vi "AlliGator Preprocess Decay v3.vi"(6 "Decay Preprocessing Parameters":T1={"Background Subtraction"=FALSE, "Straighten Decay"=FALSE, "Reverse Gates"=FALSE, "1-Normalized Decay"=FALSE, "Smoothen Decay"=FALSE, "Smoothing Parameter"=0.0, "Shift Decay"=FALSE, "Decay Shift Parameters"={"Type"=enum."Default", "Shift"=0.0, "Threshold"=0.0, "Rotate"=FALSE}, "Extrapolate Decay"=FALSE, "Additional Points"=0, "Head Fraction"=0.0, "Pixel-Normalize Decay"=FALSE, "Use Periodicity"=FALSE, "Use Cursors"=FALSE, "Tail Fraction"=0.0, "Use Decay Pre-Processing"=TRUE, "Fold Decay"=FALSE, "# Folds"=1, "[0-1]-Normalized Decay"=FALSE} {"# Folds" min=1}, 8 "Error In":errorcluster, 9 "Time-Gated Reference Decay":cluster{"t Array":dbl[], "I Array":dbl[]}, 10 "# Pixels":i32=1, 11 "Decay (in)":T9) -> (0 "Error Out":errorcluster, 3 "Decay (out)":T9, 5 "Decay Metadata":T4={"ROI Descriptor"={"Global Rectangle"=[], "Contours"=[]}, "ROI Center"={"X"=0, "Y"=0}, "Decay Background Subtraction Info"={"Laser Period"=0.0, "Gate Duration"=0.0, "Baseline Subtraction Method"=enum."Mean", "Background Definition Range"={"Min Gate"=0.0, "Max Gate"=0.0}, "Total Intensity w/o Bkgd Subtraction"=0.0, "Bkgd-subtracted Intensity (exp)"=0.0, "# Data Points"=0, "Background/Gate"=0.0, "Fitted Lifetime"=0.0, "Bkgd-subtracted Intensity (theo)"=0.0}, "Decay Reverted"=FALSE, "Decay Smoothened"=FALSE, "Decay Straightened"=FALSE, "Fitted Tau (Decay Straightening)"=0.0, "Decay Shift Parameters"={"Type"=enum."Default", "Shift"=0.0, "Threshold"=0.0, "Rotate"=FALSE}, "Decay Shifted"=FALSE, "Decay Extrapolated"=FALSE, "Decay Extrapolation Parameters"={"Additional Points"=0, "Head Fraction"=0.0, "Fitted Tau"=0.0, "Use Periodicity"=FALSE, "Use Cursors"=FALSE, "Tail Fraction"=0.0}, "Decay Normalized"=FALSE, "Fold Decay"=FALSE, "# Folds"=1} {"# Folds" min=1; "ROI Descriptor"."Contours"."Type" items=["No Selection", "Point", "Line", "Rectangle", "Oval", "Polygon", "Freehand Region", "Annulus", "Unused2", "Unused3", "Broken Line", "Freehand Line", "Rotated Rectangle"]}, 7 "Message":string)   [LabVIEW 2021, in "AlliGator Decay Analysis.lvlib" / "AlliGator Decay Preprocessing.lvlib"]
doc: "Applies the different selected pre-processing steps on the provided decay in the specified order."
uses:
  AlliGator Decay Preprocessing.lvlib
  AlliGator Decay Metadata v3.ctl
  AlliGator Decay Background Subtraction Info.ctl
  AlliGator Baseline Subtraction Method.ctl
  Graphs/XY Graph/XY Graph Plot Shift Parameters.ctl
  Graphs/XY Graph/XY Graph Plot Shift Method.ctl
  AlliGator Decay Extrapolation Parameters.ctl
  AlliGator Decay Preprocessing Parameters.ctl
  AlliGator Settings List.ctl
  AlliGator Decay Preprocessing Steps.ctl
  Variant/Variant to Data/Variant to Boolean.vi
  <vilib>/Utility/error.llb/Error Cluster From Error Code.vi
  Variant/Variant to Data/Variant to [String].vi
  <vilib>/ErrorRing/Error Ring.xnode
  AlliGator Settings.lvlib
  Variant/Variant to Data/Variant to Data.lvlib
  Graphs/XY Graph/XY Graph Add-Ons.lvlib
  AlliGator Phasor Graph.lvlib
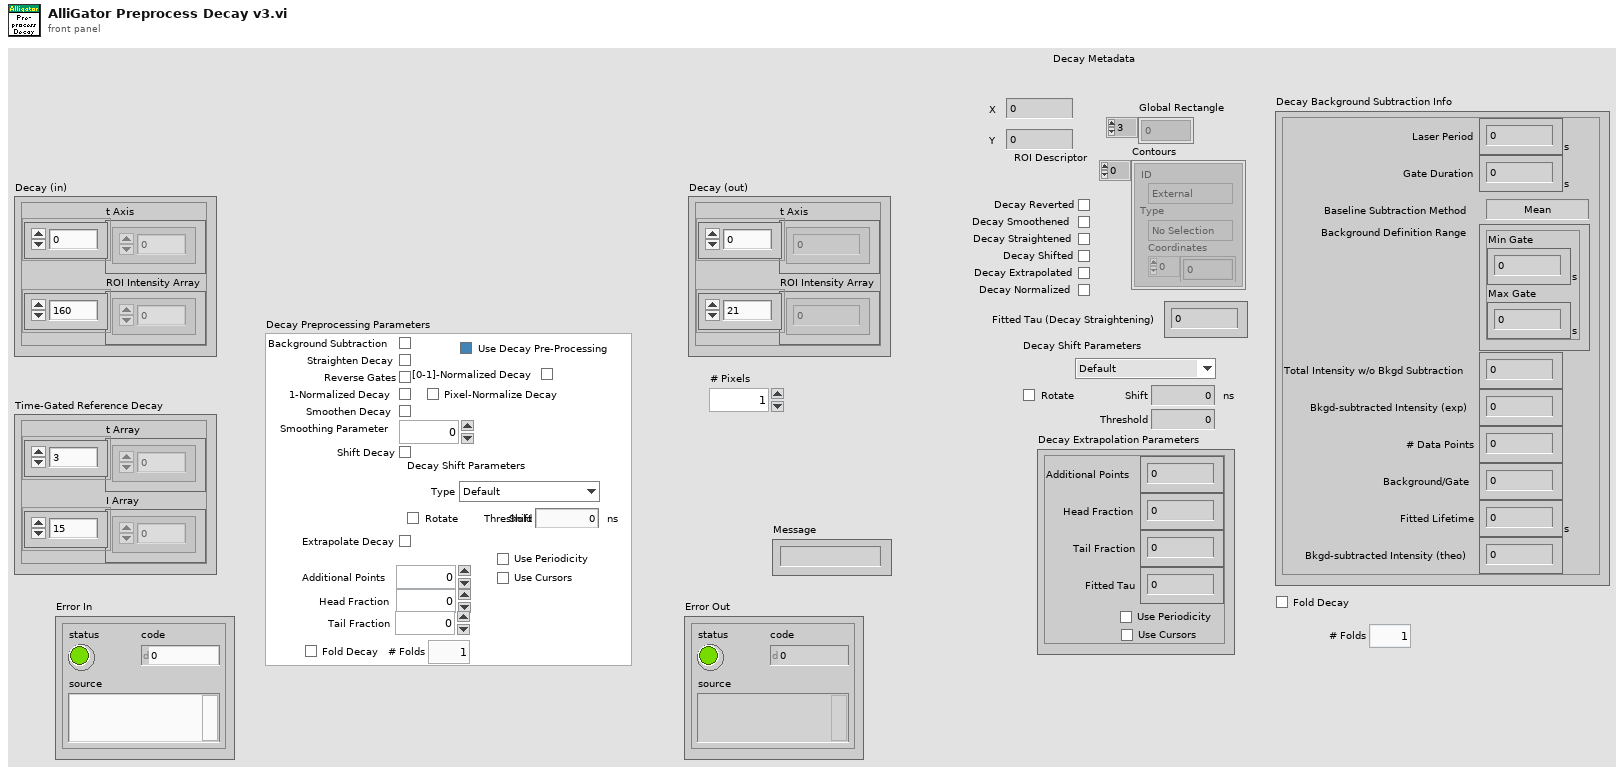
[diagram p1: front panel]
types:
  T1 = typedef "AlliGator Decay Analysis.lvlib/AlliGator Decay Preprocessing.lvlib/AlliGator Decay Preprocessing Parameters.ctl" = cluster{"Background Subtraction":bool, "Straighten Decay":bool, "Reverse Gates":bool, "1-Normalized Decay":bool, "Smoothen Decay":bool, "Smoothing Parameter":dbl, "Shift Decay":bool, "Decay Shift Parameters":T2, "Extrapolate Decay":bool, "Additional Points":u32, "Head Fraction":dbl, "Pixel-Normalize Decay":bool, "Use Periodicity":bool, "Use Cursors":bool, "Tail Fraction":dbl, "Use Decay Pre-Processing":bool, "Fold Decay":bool, "# Folds":u32, "[0-1]-Normalized Decay":bool}
  T2 = typedef "XY Graph Add-Ons.lvlib/XY Graph Plot Shift Parameters.ctl" = cluster{"Type":T3, "Shift":dbl[unit], "Threshold":dbl, "Rotate":bool}
  T3 = typedef "XY Graph Add-Ons.lvlib/XY Graph Plot Shift Method.ctl" = enum16{"Default", "CFD", "Threshold", "Cross-Correlation"}
  T4 = typedef "AlliGator Phasor Graph.lvlib/AlliGator Decay Metadata v3.ctl" = cluster{"ROI Descriptor":T5, "ROI Center":cluster{"X":i32, "Y":i32}, "Decay Background Subtraction Info":T6, "Decay Reverted":bool, "Decay Smoothened":bool, "Decay Straightened":bool, "Fitted Tau (Decay Straightening)":dbl, "Decay Shift Parameters":T2, "Decay Shifted":bool, "Decay Extrapolated":bool, "Decay Extrapolation Parameters":T8, "Decay Normalized":bool, "Fold Decay":bool, "# Folds":u32}
  T5 = typedef "ROI Descriptor" = cluster{"Global Rectangle":i32[], "Contours":cluster{"ID":enum32{"External", "Internal"}, "Type":u32, "Coordinates":i32[]}[]}
  T6 = typedef "AlliGator Decay Analysis.lvlib/AlliGator Decay Preprocessing.lvlib/AlliGator Decay Background Subtraction Info.ctl" = cluster{"Laser Period":dbl[unit], "Gate Duration":dbl[unit], "Baseline Subtraction Method":T7, "Background Definition Range":cluster{"Min Gate":dbl[unit], "Max Gate":dbl[unit]}, "Total Intensity w/o Bkgd Subtraction":dbl, "Bkgd-subtracted Intensity (exp)":dbl, "# Data Points":i32, "Background/Gate":dbl, "Fitted Lifetime":dbl[unit], "Bkgd-subtracted Intensity (theo)":dbl}
  T7 = typedef "AlliGator Decay Analysis.lvlib/AlliGator Decay Preprocessing.lvlib/AlliGator Baseline Subtraction Method.ctl" = enum16{"Mean", "Min", "Square Gated Single-Exponential", "File", "Constant"}
  T8 = typedef "AlliGator Decay Analysis.lvlib/AlliGator Decay Preprocessing.lvlib/AlliGator Decay Extrapolation Parameters.ctl" = cluster{"Additional Points":u32, "Head Fraction":dbl, "Fitted Tau":dbl, "Use Periodicity":bool, "Use Cursors":bool, "Tail Fraction":dbl}
  T9 = cluster{"t Axis":dbl[], "ROI Intensity Array":dbl[]}
  T10 = typedef "AlliGator Settings.lvlib/AlliGator Settings List.ctl" = enum16{"GUI:Visible Settings Tab", "GUI:Last Run Version", "Source Image:Use Image Histogram for Contrast", "Source Image:Low Count Pixels Rejection Options", "Source Image:High Count Pixels Rejection Options", "Source Image:Use Image Brightness", "Source Image:Blend Overlay with Image Background", "Source Image:Use Fixed ROI Diameter", "Source Image:ROI Diameter", "Source Image:ROI Center Color", "Source Image:Peak Threshold", "Source Image:Intensity Threshold", "Source Image:Image Binning Options", "Source Image:Image Smoothing Options", "Source Image:Image Histogram Active", "Source Image:Invert Binary Mask", "Source Image:Hot Pixel Removal", "Source Image:Overlay Analyzed ROI Center", "Source Image:Auto-Adjust Contrast", "Source Image:Histogram Lower Percentile", "Source Image:Histogram Upper Percentile", "Source Image:Save Source Image", "Source Image:Scale Bar Options", "Source Image:Image Resolution (Pixel Size)", "Source Image:Flatfield Correction", "Source Image:Show Dead Left Columns Correction", "Source Image:Dead Left Columns Correction", "Source Image:Image Pre-Processing Operations Order", "Data Information:Gate Width", "Data Information:Nanotime Gate Separation", "Data Information:Macrotime Gate Separation", "Data Information:Gate Step", "Data Information:# Gates", "Data Information:Gate Image Exposure", "Data Information:Gate Image Integration", "Data Information:Gates to Skip", "Data Information:Gates to Keep", "Data Information:Define Gates to", "Data Information:Channel Name", "Data Information:Available Channel Names", "Data Information:Channel Arithmetic", "Data Information:Background File Subtraction", "Data Information:Background File", "Data Information:Background Scaling Factor", "Data Information:Background Pile-up Correction", "Data Information:Background Pixel Well Capacity", "Data Information:Laser Period", "Data Information:SYNC Period", "Data Information:Pile-up Correction", "Data Information:Pixel Well Capacity", "Data Information:Dataset Scaling Factor", "Fluorescence Decay_Decay Pre-Processing:Reverse Gates", "Fluorescence Decay_Decay Pre-Processing:Verbose Decay Pre-Processing", "Fluorescence Decay_Decay Pre-Processing:Use Decay Pre-Processing", "Fluorescence Decay_Decay Pre-Processing:Background Subtraction", "Fluorescence Decay_Decay Pre-Processing:Background Definition Range", "Fluorescence Decay_Decay Pre-Processing:Baseline Subtraction Method", "Fluorescence Decay_Decay Pre-Processing:Decay Pre-Processing Operations Order", "Fluorescence Decay_Decay Pre-Processing:Smoothing Parameter", "Fluorescence Decay_Decay Pre-Processing:Shift Decay", "Fluorescence Decay_Decay Pre-Processing:Decay Shift Parameters", "Fluorescence Decay_Decay Pre-Processing:Fold Decay", "Fluorescence Decay_Decay Pre-Processing:# Folds", "Fluorescence Decay_Decay Pre-Processing:1-Normalize Decay", "Fluorescence Decay_Decay Pre-Processing:[0-1]-Normalize Decay", "Fluorescence Decay_Decay Pre-Processing:Smoothen Decay", "Fluorescence Decay_Decay Pre-Processing:Extrapolate Decay", "Fluorescence Decay_Decay Pre-Processing:Use Periodicity", "Fluorescence Decay_Decay Pre-Processing:Use Cursors", "Fluorescence Decay_Decay Pre-Processing:Tail Fraction", "Fluorescence Decay_Decay Pre-Processing:Head Fraction", "Fluorescence Decay_Decay Pre-Processing:Additional Points", "Fluorescence Decay_Decay Pre-Processing:Straighten Decay", "Fluorescence Decay_Decay Pre-Processing:Constant Background", "Fluorescence Decay_Decay Pre-Processing:Pixel-Normalize Decay", "Fluorescence Decay_Advanced Analysis:Extract IRF instead of Decay", "Fluorescence Decay_Advanced Analysis:IRF Extraction Options", "Fluorescence Decay_Advanced Analysis:IRF Optimization Options", "Fluorescence Decay_Advanced Analysis:Square Pulse Options", "Fluorescence Decay_Advanced Analysis:IRF Order", "Fluorescence Decay_Advanced Analysis:IRF Time Constants", "Fluorescence Decay_Advanced Analysis:Wavelet Analysis Options", "Fluorescence Decay_Advanced Analysis:Average Lifetime Options", "Fluorescence Decay_Fit Options:Fit Options", "Fluorescence Decay_Fit Options:Use Legacy Fitting Approach", "Fluorescence Decay_Fit Options:Use Data Information Laser Period", "Fluorescence Decay_Fit Parameters:Displayed Fit Parameters", "Fluorescence Decay_Fit Parameters:Fit Parameter Constraints", "Fluorescence Decay_Fit Parameters:Export Tabulated Results", "Fluorescence Decay_Fit Parameters:MLE Baseline Offset Type", "Fluorescence Decay_Fit Parameters:MLE Baseline Offset", "Fluorescence Decay_Fit Parameters:Guess Parameter Names", "Fluorescence Decay_Fit Parameters:Guess Parameter Values", "Fluorescence Decay_Fit Parameters:Guess Parameters Options", "Fluorescence Decay_Styles:Show Last Decay Only", "Fluorescence Decay_Styles:Decay Graph Color Array", "Fluorescence Decay:Decay Graph Active", "Fluorescence Decay Statistics:Min Peak Value", "Fluorescence Decay Statistics:Reject Low Decay Peak Pixels", "Fluorescence Decay Statistics:Reject High Decay Peak Pixels", "Fluorescence Decay Statistics:Max Peak Value", "Time Traces:Use File Timestamp", "Time Traces:Time Step", "Time Traces:Use Intensity Correction File", "Time Traces:Intensity Correction File", "Phasor Plot:Phasor Plot Smoothing Options", "Phasor Plot:Phasor Plot Size", "Phasor Plot:Phasor Plot Graphics Options", "Phasor Plot:Cumulative Phasor Plot", "Phasor Plot:Use Phasor Brightness", "Phasor Plot:Blend Overlay with Phasor Background", "Phasor Plot:Save Phasor Plot", "Phasor Plot:Show References", "Phasor Plot:Phasor Ratio Decay Range", "Phasor Plot:Exponential Fading", "Phasor Plot:Phasor Ratio Reference Colors", "Phasor Plot:Reference Radius", "Phasor Plot:Show Color Map Vertices", "Phasor Plot:Phasor Plot Active", "Phasor Plot:Phasor Ratio Color Map Type", "Phasor Plot:Phasor Ratio Color Map", "Phasor Plot:Phasor Ratio Display Range", "Phasor Plot:Selected Image ROI(s)", "Phasor Plot:All Image ROIs", "Phasor Plot:Selected Phasor Plot ROI(s)", "Phasor Plot:All Phasor Plot ROIs", "Phasor Plot:Phasor Ratio Color-Coded Quantity", "Phasor Plot:Store Phasor Harmonics", "Phasor Plot:Draw Reference Segment", "Phasor Plot:User-Defined Quantity", "Phasor Graph:Phasor Frequency", "Phasor Graph:Phasor Ratio Type", "Phasor Graph:Pixel-level Phasor Computation", "Phasor Graph:Save Phasor Graph", "Phasor Graph:Phasor Graph Active", "Phasor Graph:Phasor SDV Options", "Phasor Calibration:Use Backup Calibration if needed", "Phasor Graph:Define Shortest Lifetime as", "Phasor Calibration:Backup Calibration Type", "Phasor Calibration:Calibration Type", "Phasor Calibration:Calibration Lifetime", "Phasor Calibration:Calibration Map Algorithm", "Single-Exponential Phasor Locus (SEPL):Gate Parameters", "Single-Exponential Phasor Locus (SEPL):User-defined Gate", "Single-Exponential Phasor Locus (SEPL):User-defined IRF", "Single-Exponential Phasor Locus (SEPL):Phasor Parameters", "Single-Exponential Phasor Locus (SEPL):Decay & IRF Parameters", "Single-Exponential Phasor Locus (SEPL):Display Parameters", "Lifetime Analysis:Decay Analysis Parameters", "Lifetime Analysis:Lifetime Map Active", "Plugins:Python Settings", "Miscellaneous:Verbose Mode", "Miscellaneous:Beep after Script", "Miscellaneous:Saved Image File Format", "Miscellaneous:Exported Gate Image Settings", "Miscellaneous:Include Loading in Timing", "Miscellaneous:Verbose Settings Mode", "Miscellaneous:Histogram Options", "Miscellaneous:Beep on Error", "Miscellaneous:# Logical Processors Used", "Miscellaneous:ROI Description Max Characters", "Miscellaneous:Verbose Error Mode", "Miscellaneous:Transparent Mask Color"}
  T11 = typedef "AlliGator Phasor Graph.lvlib/AlliGator Decay Preprocessing Steps.ctl" = enum16{"Reverse Decay", "Smooth Decay", "Straighten Decay", "Shift/Rotate Decay", "Extrapolate Decay", "Normalize Decay"}
  T12 = cluster{"t Axis":dbl[], "ROI Intensity Array in":dbl[]}
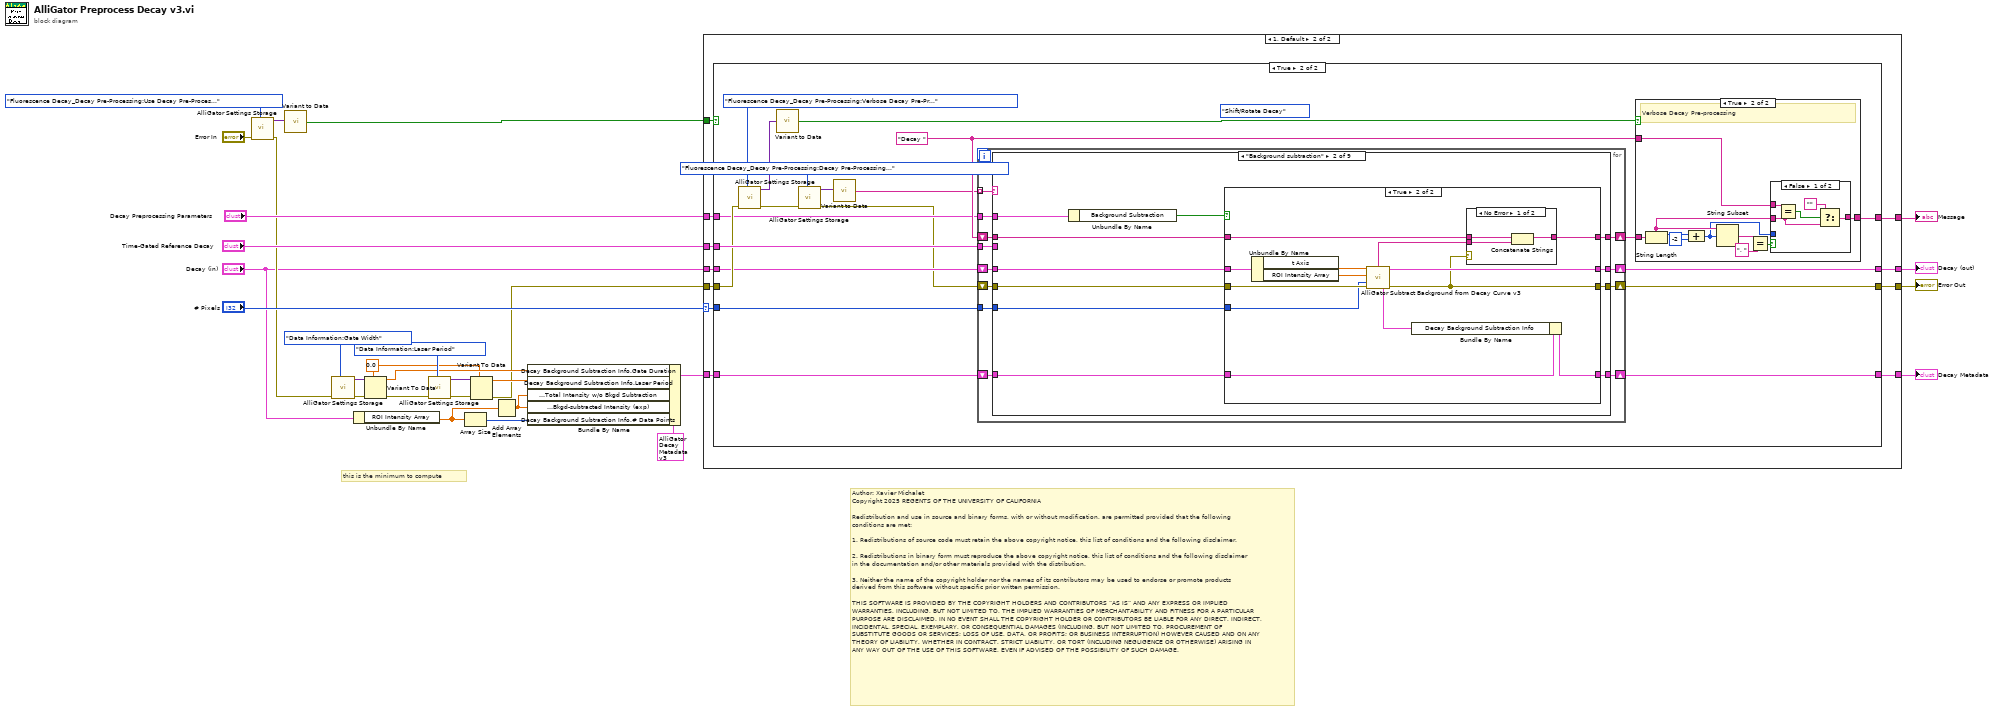
[diagram p0: block diagram]
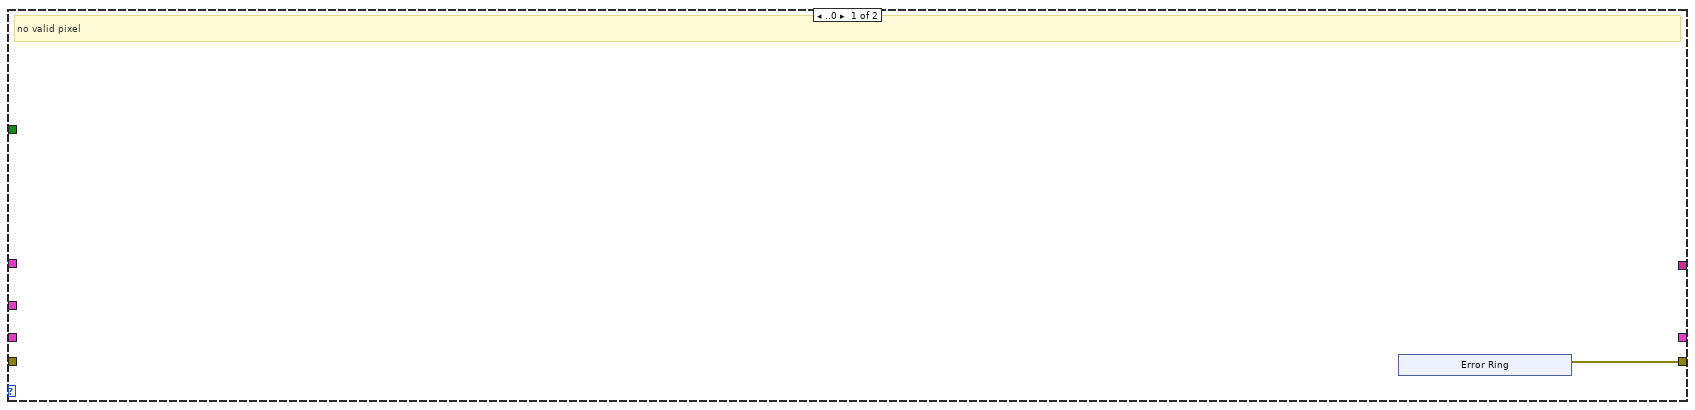
[diagram p2: hidden frame]
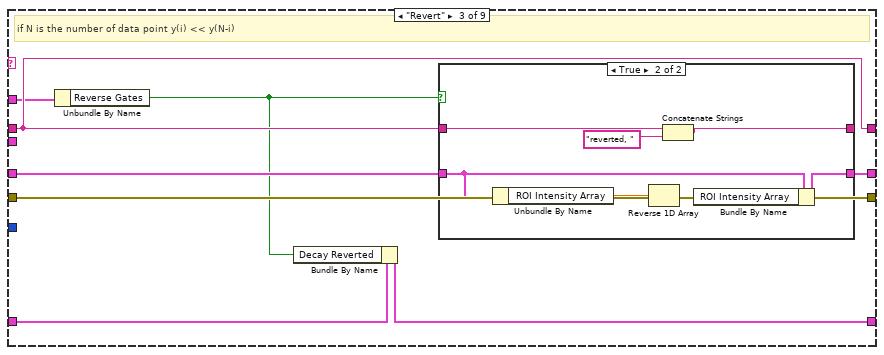
[diagram p7: hidden frame]
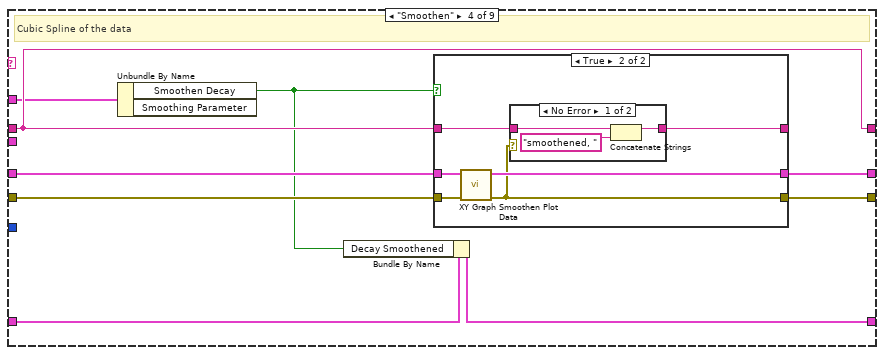
[diagram p9: hidden frame]
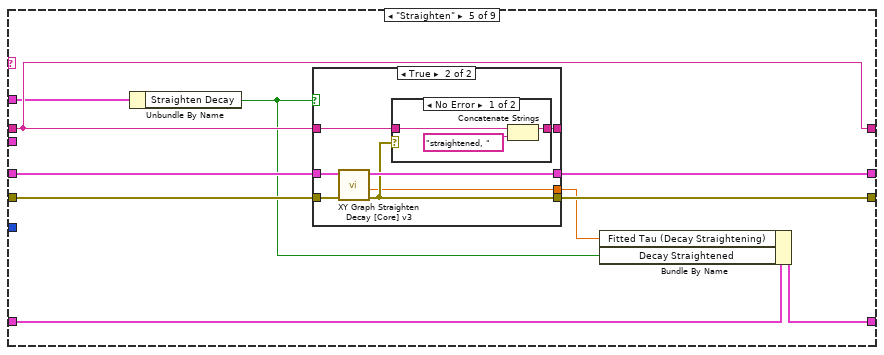
[diagram p12: hidden frame]
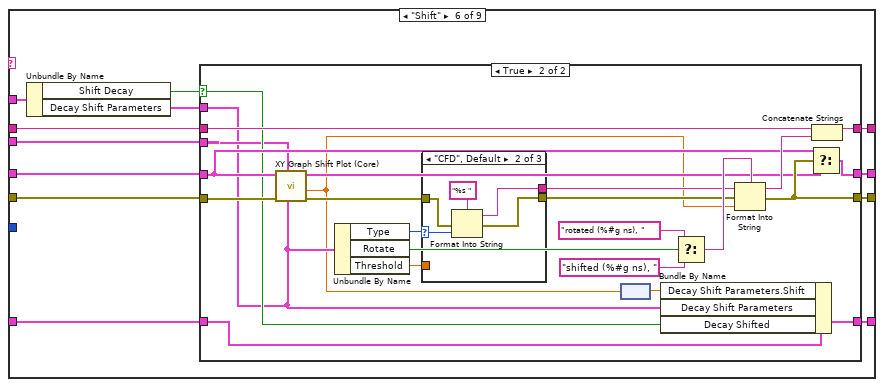
[diagram p15: hidden frame]
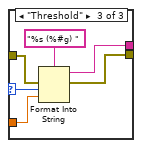
[diagram p18: hidden frame]
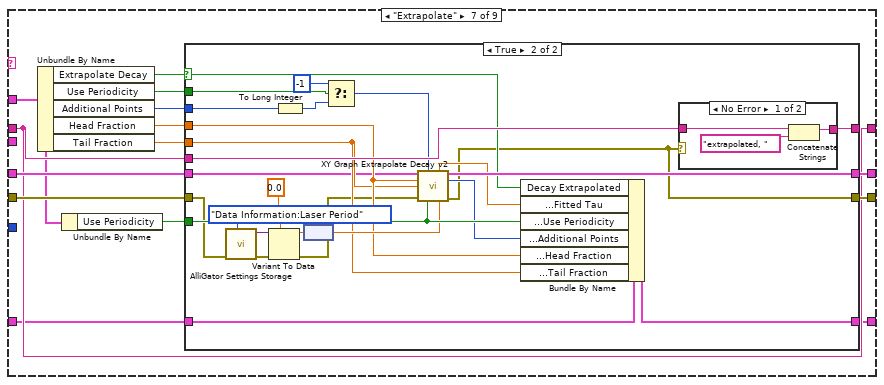
[diagram p19: hidden frame]
diagram:
  w1 = dbl[unit] 0.0 ("Min Gate")
  # "Author: Xavier Michalet\nCopyright 2025 REGENTS OF THE UNIVERSITY OF CALIFORNIA\n\nRedistribution and use in source and binary forms, with or without modification, are permitted provided that the following conditions are met:\n\n1. Redistributions of source code must retain the above copyright notice, this list of conditions and the following disclaimer.\n\n2. Redistributions in binary form must reproduce the above copyright notice, this list of conditions and the following disclaimer in the documentation and/or other materials provided with the distribution.\n\n3. Neither the name of the copyright holder nor the names of its contributors may be used to endorse or promote products derived from this software without specific prior written permission.\n\nTHIS SOFTWARE IS PROVIDED BY THE COPYRIGHT HOLDERS AND CONTRIBUTORS “AS IS” AND ANY EXPRESS OR IMPLIED WARRANTIES, INCLUDING, BUT NOT LIMITED TO, THE IMPLIED WARRANTIES OF MERCHANTABILITY AND FITNESS FOR A PARTICULAR PURPOSE ARE DISCLAIMED. IN NO EVENT SHALL THE COPYRIGHT HOLDER OR CONTRIBUTORS BE LIABLE FOR ANY DIRECT, INDIRECT, INCIDENTAL, SPECIAL, EXEMPLARY, OR CONSEQUENTIAL DAMAGES (INCLUDING, BUT NOT LIMITED TO, PROCUREMENT OF SUBSTITUTE GOODS OR SERVICES; LOSS OF USE, DATA, OR PROFITS; OR BUSINESS INTERRUPTION) HOWEVER CAUSED AND ON ANY THEORY OF LIABILITY, WHETHER IN CONTRACT, STRICT LIABILITY, OR TORT (INCLUDING NEGLIGENCE OR OTHERWISE) ARISING IN ANY WAY OUT OF THE USE OF THIS SOFTWARE, EVEN IF ADVISED OF THE POSSIBILITY OF SUCH DAMAGE."
  # "this is the minimum to compute"
  n1 = call "AlliGator Settings Storage.vi"("AlliGator Settings List"=AlliGator_Settings_List."Fluorescence Decay_Decay Pre-Processing:Use Decay Pre-Processing", "Error In"="Error In") -> ("Error Out"=w6:errorcluster, "Variant Data out"=w23:variant)  [unwired: 8 in]
  n2 = call-poly "Variant to Data.vi"("Variant"=w23) -> ("Value"=w20:bool)  [unwired: 8 in]
  n3 = call "AlliGator Settings Storage.vi"("AlliGator Settings List"=AlliGator_Settings_List."Data Information:Gate Width", "Error In"=w6) -> ("Error Out"=w15:errorcluster, "Variant Data out"=w16:variant)  [unwired: 8 in]
  n4 = Unbundle By Name("Decay (in)") -> ("ROI Intensity Array"=w18:dbl[])
  n5 = Variant To Data(error in=w15, type=w1, Variant=w16) -> (data=w10:dbl[unit], error out=w7:errorcluster)
  n6 = call "AlliGator Settings Storage.vi"("AlliGator Settings List"=AlliGator_Settings_List."Data Information:Laser Period", "Error In"=w7) -> ("Error Out"=w14:errorcluster, "Variant Data out"=w13:variant)  [unwired: 8 in]
  n7 = Array Size(array=w18) -> (size(s)=w17:i32)
  n8 = Variant To Data(error in=w14, type=w1, Variant=w13) -> (data=w11:dbl[unit], error out=w5:errorcluster)
  n9 = Add Array Elements(numeric array=w18) -> (sum=w9:dbl)
  n10 = Bundle By Name(cluster=T4 {"ROI Descriptor"={"Global Rectangle"=[], "Contours"=[]}, "ROI Center"={"X"=0, "Y"=0}, "Decay Background Subtraction Info"={"Laser Period"=0.0, "Gate Duration"=0.0, "Baseline Subtraction Method"=enum."Mean", "Background Definition Range"={"Min Gate"=0.0, "Max Gate"=0.0}, "Total Intensity w/o Bkgd Subtraction"=0.0, "Bkgd-subtracted Intensity (exp)"=0.0, "# Data Points"=0, "Background/Gate"=0.0, "Fitted Lifetime"=0.0, "Bkgd-subtracted Intensity (theo)"=0.0}, "Decay Reverted"=FALSE, "Decay Smoothened"=FALSE, "Decay Straightened"=FALSE, "Fitted Tau (Decay Straightening)"=0.0, "Decay Shift Parameters"={"Type"=enum."Default", "Shift"=0.0, "Threshold"=0.0, "Rotate"=FALSE}, "Decay Shifted"=FALSE, "Decay Extrapolated"=FALSE, "Decay Extrapolation Parameters"={"Additional Points"=0, "Head Fraction"=0.0, "Fitted Tau"=0.0, "Use Periodicity"=FALSE, "Use Cursors"=FALSE, "Tail Fraction"=0.0}, "Decay Normalized"=FALSE, "Fold Decay"=FALSE, "# Folds"=1} ("Decay Metadata"), "Decay Background Subtraction Info.Gate Duration"=w10, "Decay Background Subtraction Info.Laser Period"=w11, "Decay Background Subtraction Info.Total Intensity w/o Bkgd Subtraction"=w9, "Decay Background Subtraction Info.Bkgd-subtracted Intensity (exp)"=w9, "Decay Background Subtraction Info.# Data Points"=w17) -> (w4:T4)
  n11 = case shown="1, Default" "# Pixels" {
    selector: "# Pixels" -> [_ w40]
    tunnel: [_ w45] -> w29
    tunnel: [_ w44] -> w28
    tunnel: "Time-Gated Reference Decay" -> [_ w43]
    tunnel: [w30 w42] -> w26
    tunnel: [_ w41] -> w25
    tunnel: w20 -> [_ w39]
    tunnel: "Decay Preprocessing Parameters" -> [_ w38]
    tunnel: w5 -> [_ w37]
    tunnel: w4 -> [_ w36]
    tunnel: "Decay (in)" -> [_ w35]
    frame ..0 {
      # "no valid pixel"
      n12 = xnode "Error Ring"() -> ("error out"=w30:errorcluster)
    }
    frame 1, Default {
      n13 = case shown="True" w39 {
        tunnel: [_ w68] -> w45
        tunnel: [w48 w67] -> w44
        tunnel: w43 -> [_ w66]
        tunnel: [w47 w64] -> w42
        tunnel: w35 -> [w48 w52]
        tunnel: [w46 w61] -> w41
        tunnel: w40 -> [_ w50]
        tunnel: w37 -> [w47 w54]
        tunnel: w38 -> [_ w53]
        tunnel: w36 -> [w46 w49]
        frame False {
        }
        frame True {
          (unwired) AlliGator_Decay_Preprocessing_Steps."Shift/Rotate Decay" ("Preprocessing Operations Order")
          w60 = "Decay " ("Message")
          n14 = call "AlliGator Settings Storage.vi"("AlliGator Settings List"=AlliGator_Settings_List."Fluorescence Decay_Decay Pre-Processing:Verbose Decay Pre-Processing", "Error In"=w54) -> ("Error Out"=w55:errorcluster, "Variant Data out"=w59:variant)  [unwired: 8 in]
          n15 = call-poly "Variant to Data.vi"("Variant"=w59) -> ("Value"=w57:bool)  [unwired: 8 in]
          n16 = call "AlliGator Settings Storage.vi"("AlliGator Settings List"=AlliGator_Settings_List."Fluorescence Decay_Decay Pre-Processing:Decay Pre-Processing Operations Order", "Error In"=w55) -> ("Error Out"=w51:errorcluster, "Variant Data out"=w62:variant)  [unwired: 8 in]
          n17 = call-poly "Variant to Data.vi"("Variant"=w62) -> ("String Array"=w56:string[])  [unwired: 8 in]
          n18 = for {
            shift-right: [w79] -> w67
            shift-left: w52 -> [w80]
            shift-right: [w69] -> w65
            shift-left: w60 -> [w78]
            shift-right: [w76] -> w64
            shift-left: w51 -> [w77]
            tunnel: w66 -> [w75]
            tunnel: w56 -> [w74] mode=indexing
            shift-right: [w73] -> w61
            shift-left: w49 -> [w72]
            tunnel: w50 -> [w71]
            tunnel: w53 -> [w70]
            n19 = case shown="\"Background subtraction\"" w74 {
              tunnel: w80 -> [w84 w94 w123 w141 w163 w189 w243 w290 w324]
              tunnel: [w84 w93 w122 w140 w162 w188 w242 w289 w323] -> w79
              tunnel: [w81 w90 w121 w138 w164 w185 w239 w280 w317] -> w69
              tunnel: w78 -> [w81 w90 w121 w138 w164 w185 w239 w291 w325]
              tunnel: w77 -> [w83 w92 w120 w139 w161 w186 w241 w288 w322]
              tunnel: [w83 w91 w120 w137 w160 w187 w240 w287 w321] -> w76
              tunnel: w75 -> [_ _ _ _ _ w184 _ _ _]
              tunnel: [w82 w89 w118 w135 w157 w183 w237 w285 w319] -> w73
              tunnel: w72 -> [w82 w88 w119 w136 w159 w182 w238 w286 w320]
              tunnel: w71 -> [_ w85 _ _ _ _ _ w282 _]
              tunnel: w70 -> [_ w86 w116 w133 w155 w179 w230 w281 w316]
              frame Default {
              }
              frame "Background subtraction" {
                n20 = Unbundle By Name(w86) -> ("Background Subtraction"=w87:bool)
                n21 = case shown="True" w87 {
                  tunnel: w94 -> [w97 w111]
                  tunnel: [w97 w107] -> w93
                  tunnel: w92 -> [w98 w108]
                  tunnel: [w98 w106] -> w91
                  tunnel: w90 -> [w96 w105]
                  tunnel: [w96 w104] -> _
                  tunnel: [w95 w100] -> w89
                  tunnel: w88 -> [w95 w101]
                  tunnel: w85 -> [_ w99]
                  frame False {
                  }
                  frame True {
                    n22 = Unbundle By Name(w111) -> ("t Axis"=w110:dbl[], "ROI Intensity Array"=w109:dbl[])
                    n23 = call "AlliGator Subtract Background from Decay Curve v3.vi"("t Axis"=w110, "ROI Intensity Array in"=w109, "# ROI Pixels (1)"=w99, "Error In"=w108) -> ("Decay (out)"=w107:T12, "Message"=w103:string, "Decay Background Subtraction Info"=w102:T6, "Error Out"=w106:errorcluster)  [unwired: 4 in, 4 out]
                    n24 = Bundle By Name(cluster=w101, "Decay Background Subtraction Info"=w102) -> (w100:T4)
                    n25 = case shown="No Error" w106 {
                      tunnel: w105 -> [w114 w115]
                      tunnel: [w112 w115] -> w104
                      tunnel: w103 -> [w113 _]
                      frame No Error {
                        n26 = Concatenate Strings(w114, w113) -> (w112:string)
                      }
                      frame Error {
                      }
                    }
                  }
                }
              }
              frame "Revert" {
                # "if N is the number of data point y(i) << y(N-i)"
                n27 = Unbundle By Name(w116) -> ("Reverse Gates"=w117:bool)
                n28 = Bundle By Name(cluster=w119, "Decay Reverted"=w117) -> (w118:T4)
                n29 = case shown="True" w117 {
                  tunnel: w123 -> [w125 w132]
                  tunnel: [w125 w131] -> w122
                  tunnel: [w124 w126] -> _
                  tunnel: w121 -> [w124 w128]
                  frame False {
                  }
                  frame True {
                    n30 = Unbundle By Name(w132) -> ("ROI Intensity Array"=w130:dbl[])
                    n31 = Reverse 1D Array(array=w130) -> (reversed array=w129:dbl[])
                    n32 = Concatenate Strings(w128, "reverted, " ("Message")) -> (w126:string)
                    n33 = Bundle By Name(cluster=w132, "ROI Intensity Array"=w129) -> (w131:T9)
                  }
                }
              }
              frame "Smoothen" {
                # "Cubic Spline of the data"
                n34 = Unbundle By Name(w133) -> ("Smoothen Decay"=w134:bool)  [unwired: 1 out]
                n35 = Bundle By Name(cluster=w136, "Decay Smoothened"=w134) -> (w135:T4)
                n36 = case shown="True" w134 {
                  tunnel: w141 -> [w144 w150]
                  tunnel: [w144 w149] -> w140
                  tunnel: w139 -> [w143 w148]
                  tunnel: [w143 w145] -> w137
                  tunnel: w138 -> [w142 w146]
                  tunnel: [w142 w147] -> _
                  frame False {
                  }
                  frame True {
                    n37 = call "XY Graph Smoothen Plot Data.vi"("Error In"=w148, "Plot"=w150) -> ("error out"=w145:errorcluster, "Cubic Splined Plot"=w149:cluster{"X Array":dbl[], "Y Array":dbl[]})  [unwired: 8 in]
                    n38 = case shown="No Error" w145 {
                      tunnel: [w153 w154] -> w147
                      tunnel: w146 -> [w151 w154]
                      frame No Error {
                        n39 = Concatenate Strings(w151, "smoothened, " ("string")) -> (w153:string)
                      }
                      frame Error {
                      }
                    }
                  }
                }
              }
              frame "Straighten" {
                n40 = Unbundle By Name(w155) -> ("Straighten Decay"=w156:bool)
                n41 = case shown="True" w156 {
                  tunnel: w163 -> [w167 w174]
                  tunnel: w161 -> [w166 w173]
                  tunnel: [w167 w172] -> w162
                  tunnel: [w166 w169] -> w160
                  tunnel: w164 -> [w165 w171]
                  tunnel: [w165 w170] -> _
                  tunnel: [_ w168] -> w158
                  frame False {
                  }
                  frame True {
                    n42 = call "XY Graph Straighten Decay [Core] v3.vi"("Error In"=w173, "Plot in"=w174) -> ("error out"=w169:errorcluster, "Fitted Tau"=w168:dbl, "Plot out"=w172:cluster{"X Array":dbl[], "Y Array":dbl[]})  [unwired: 7 in]
                    n43 = case shown="No Error" w169 {
                      tunnel: w171 -> [w177 w178]
                      tunnel: [w176 w178] -> w170
                      frame No Error {
                        n44 = Concatenate Strings(w177, "straightened, " ("string")) -> (w176:string)
                      }
                      frame Error {
                      }
                    }
                  }
                }
                n45 = Bundle By Name(cluster=w159, "Fitted Tau (Decay Straightening)"=w158, "Decay Straightened"=w156) -> (w157:T4)
              }
              frame "Shift" {
                n46 = Unbundle By Name(w179) -> ("Shift Decay"=w181:bool, "Decay Shift Parameters"=w180:T2)
                n47 = case shown="True" w181 {
                  selector: w181 -> [_ w205]
                  tunnel: w180 -> [_ w201]
                  tunnel: w184 -> [_ w202]
                  tunnel: w189 -> [w193 w207]
                  tunnel: [w193 w208] -> w188
                  tunnel: w186 -> [w192 w212]
                  tunnel: [w192 w210] -> w187
                  tunnel: w185 -> [w191 w211]
                  tunnel: [w191 w217] -> _
                  tunnel: [w190 w206] -> w183
                  tunnel: w182 -> [w190 w200]
                  frame False {
                  }
                  frame True {
                    n48 = call "XY Graph Shift Plot (Core).vi"("Plot Shift Parameters"=w201, "Time-Gated Reference Decay"=w202, "error in (no error)"=w212, "Decay in"=w207) -> ("error out"=w197:errorcluster, "Shift (ns)"=w194:dbl, "Decay out"=w209:T12)  [unwired: 5 in]
                    n49 = Unbundle By Name(w201) -> ("Type"=w199:T3, "Rotate"=w203:bool, "Threshold"=w195:dbl)
                    n50 = case shown="\"CFD\", Default" w199 {
                      selector: w199 -> [_ w223 w229]
                      tunnel: [_ w219 w225] -> w198
                      tunnel: w197 -> [w218 w221 w227]
                      tunnel: [w218 w220 w226] -> w196
                      tunnel: w195 -> [_ _ w224]
                      frame "Default" {
                      }
                      frame "CFD", Default {
                        n51 = Format Into String(format string="%s ", error in=w221, w223) -> (resulting string=w219:string, error out=w220:errorcluster)  [unwired: 1 in]
                      }
                      frame "Threshold" {
                        n52 = Format Into String(format string="%s (%#g) ", error in=w227, w229, w224) -> (resulting string=w225:string, error out=w226:errorcluster)  [unwired: 1 in]
                      }
                    }
                    n53 = node(w194) -> (w204:dbl[unit])
                    n54 = Bundle By Name(cluster=w200, "Decay Shift Parameters.Shift"=w204, "Decay Shift Parameters"=w201, "Decay Shifted"=w205) -> (w206:T4)
                    n55 = Select(t="rotated (%#g ns), " ("string"), s=w203, f="shifted (%#g ns), " ("string")) -> (s? t:f=w213:string)
                    n56 = Format Into String(format string=w213, initial string=w198, error in=w196, w194) -> (resulting string=w214:string, error out=w210:errorcluster)
                    n57 = Select(t=w207, s=w210, f=w209) -> (s? t:f=w208:T12)
                    n58 = Concatenate Strings(w211, w214) -> (w217:string)
                  }
                }
              }
              frame "Extrapolate" {
                n59 = Unbundle By Name(w230) -> ("Extrapolate Decay"=w232:bool, "Use Periodicity"=w231:bool, "Additional Points"=w235:u32, "Head Fraction"=w236:dbl, "Tail Fraction"=w233:dbl)
                n60 = Unbundle By Name(w230) -> ("Use Periodicity"=w234:bool)
                n61 = case shown="True" w232 {
                  selector: w232 -> [_ w259]
                  tunnel: w243 -> [w247 w256]
                  tunnel: [w247 w273] -> w242
                  tunnel: w241 -> [w246 w250]
                  tunnel: [w246 w255] -> w240
                  tunnel: w239 -> [w245 w272]
                  tunnel: [w245 w271] -> _
                  tunnel: w235 -> [_ w260]
                  tunnel: w236 -> [_ w258]
                  tunnel: w238 -> [w244 w269]
                  tunnel: [w244 w270] -> w237
                  tunnel: w234 -> [_ w268]
                  tunnel: w233 -> [_ w257]
                  tunnel: w231 -> [_ w262]
                  frame False {
                  }
                  frame True {
                    n62 = call "AlliGator Settings Storage.vi"("AlliGator Settings List"=AlliGator_Settings_List."Data Information:Laser Period", "Error In"=w250) -> ("Error Out"=w252:errorcluster, "Variant Data out"=w253:variant)  [unwired: 8 in]
                    n63 = Variant To Data(error in=w252, type=dbl[unit] 0.0 ("Decay Extrapolation Parameters.Fitted Tau"), Variant=w253) -> (data=w248:dbl[unit], error out=w251:errorcluster)
                    n64 = To Long Integer(number=w260) -> (32bit integer=w263:i32)
                    n65 = node(w248) -> (w267:dbl)
                    n66 = Select(t=-1, s=w262, f=w263) -> (s? t:f=w261:i32)
                    n67 = call "XY Graph Extrapolate Decay v2.vi"("Plot in"=w256, "# Additional Points (-1: to Period)"=w261, "Head Fraction"=w258, "Tail Fraction"=w257, "Error In"=w251, "Periodic Decay"=w268, "Period"=w267) -> ("Fitted Tau"=w266:dbl, "Plot out"=w273:cluster{"X Array":dbl[], "Y Array":dbl[]}, "# Additional Points"=w265:i32, "error out"=w255:errorcluster)  [unwired: 3 in, 2 out]
                    n68 = Bundle By Name(cluster=w269, "Decay Extrapolated"=w259, "Decay Extrapolation Parameters.Fitted Tau"=w266, "Decay Extrapolation Parameters.Use Periodicity"=w268, "Decay Extrapolation Parameters.Additional Points"=w265, "Decay Extrapolation Parameters.Head Fraction"=w258, "Decay Extrapolation Parameters.Tail Fraction"=w257) -> (w270:T4)
                    n69 = case shown="No Error" w255 {
                      tunnel: w272 -> [w276 w277]
                      tunnel: [w275 w277] -> w271
                      frame No Error {
                        n70 = Concatenate Strings(w276, "extrapolated, " ("string")) -> (w275:string)
                      }
                      frame Error {
                      }
                    }
                  }
                }
              }
              frame "Normalize" {
                n71 = Unbundle By Name(w281) -> ("1-Normalized Decay"=w279:bool, "[0-1]-Normalized Decay"=w278:bool, "Pixel-Normalize Decay"=w283:bool)
                n72 = Compound Arithmetic op=OR(w279, w278, w283) -> (w284:bool)
                n73 = case shown="True" w284 {
                  tunnel: w290 -> [w294 w306]
                  tunnel: [w294 w311] -> w289
                  tunnel: w288 -> [w293 w310]
                  tunnel: [w293 w307] -> w287
                  tunnel: [w292 w309] -> w280
                  tunnel: w291 -> [w292 w308]
                  tunnel: w283 -> [_ w301]
                  tunnel: w282 -> [_ w305]
                  tunnel: w278 -> [_ w299]
                  frame False {
                  }
                  frame True {
                    n74 = Compound Arithmetic op=AND(w299, invert w301) -> (w302:bool)
                    n75 = Select(t=w305, s=w301, f=nan) -> (s? t:f=w304:dbl)
                    n76 = Select(t="[0, 1]-normalized, " ("string"), s=w299, f="1-normalized, " ("string")) -> (s? t:f=w296:string)
                    n77 = call "XY Graph Normalize Plot.vi"("Error In"=w310, "Normalization Factor (Max *)"=w304, "Subtract Baseline? (No)"=w302, "Plot in"=w306) -> ("Error Out"=w307:errorcluster, "Plot out"=w311:cluster{"X Array":dbl[], "Y Array":dbl[]})  [unwired: 6 in]
                    n78 = Select(t="pixel-normalized, " ("string"), s=w301, f=w296) -> (s? t:f=w295:string)
                    n79 = case shown="No Error" w307 {
                      tunnel: [w314 w315] -> w309
                      tunnel: w308 -> [w313 w315]
                      tunnel: w295 -> [w312 _]
                      frame No Error {
                        n80 = Concatenate Strings(w313, w312) -> (w314:string)
                      }
                      frame Error {
                      }
                    }
                  }
                }
                n81 = Bundle By Name(cluster=w286, "Decay Normalized"=w284) -> (w285:T4)
              }
              frame "Fold" {
                n82 = Unbundle By Name(w316) -> ("Fold Decay"=w328:bool, "# Folds"=w318:u32)
                n83 = Decrement(x=w318) -> (x-1=w329:u32)
                n84 = Not Equal To 0?(x=w329) -> (x != 0?=w327:bool)
                n85 = And(x=w328, y=w327) -> (x .and. y?=w326:bool)
                n86 = case shown="True" w326 {
                  tunnel: w325 -> [w330 w334]
                  tunnel: [w330 w335] -> w317
                  tunnel: w324 -> [w333 w337]
                  tunnel: [w333 w336] -> w323
                  tunnel: w322 -> [w332 w339]
                  tunnel: [w332 w338] -> w321
                  tunnel: w320 -> [w331 w343]
                  tunnel: [w331 w340] -> w319
                  tunnel: w318 -> [_ w342]
                  frame False {
                  }
                  frame True {
                    n87 = Bundle By Name(cluster=w343, "Fold Decay"=TRUE, "# Folds"=w342) -> (w340:T4)
                    n88 = call "XY Graph Fold Plot xn.vi"("Error In"=w339, "Message in"=w334, "# Folds"=w342, "Decay (in) in"=w337) -> ("Error Out"=w338:errorcluster, "Message out"=w335:string, "Decay (in) out"=w336:cluster{"X Axis":dbl[], "Y Axis":dbl[]})  [unwired: 4 in, 1 out]
                  }
                }
              }
            }
          }
          n89 = case shown="True" w57 {
            tunnel: [_ w348] -> w68
            tunnel: w65 -> [_ w347]
            tunnel: w60 -> [_ w346]
            frame False {
              # "Silent Decay Pre-processing"
            }
            frame True {
              # "Verbose Decay Pre-processing"
              n90 = String Length(string=w347) -> (length=w352:i32)
              n91 = Compound Arithmetic op=ADD(w352, -2 ("value")) -> (w345:i32)
              n92 = String Subset(string=w347, offset (0)=w345) -> (substring=w351:string)  [unwired: 1 in]
              n93 = Equal?(x=w351, y=", ") -> (x = y?=w349:bool)
              n94 = case shown="False" w349 {
                tunnel: [w354 w359] -> w348
                tunnel: w347 -> [w356 w360]
                tunnel: w345 -> [_ w358]
                tunnel: w346 -> [w357 _]
                frame False {
                  n95 = Equal?(x=w357, y=w356) -> (x = y?=w353:bool)
                  n96 = Select(t="", s=w353, f=w356) -> (s? t:f=w354:string)
                }
                frame True {
                  n97 = String Subset(string=w360, length (rest)=w358) -> (substring=w359:string)  [unwired: 1 in]
                }
              }
            }
          }
        }
      }
    }
  }
  "Decay (out)" <- w28
  "Error Out" <- w26
  "Message" <- w29
  "Decay Metadata" <- w25
